vi "EditValue.vi"(8 "error in (no error)":errorcluster, 10 "Bounds":T1, 11 "Floating point base in":refnum<class "Floating point base.lvclass">) -> (0 "error out":errorcluster, 1 "Tabbed out?":bool, 2 "Value changed?":bool, 3 "Floating point base out":refnum<class "Floating point base.lvclass">)   [LabVIEW 2018, in "D Datagrid Library.lvlib" / "Floating point base.lvclass"]
uses:
  Floating point base.lvclass
  <vilib>/Utility/miscctls.llb/LVRectTypeDef.ctl
  DatagridElement/DatagridElement.lvclass
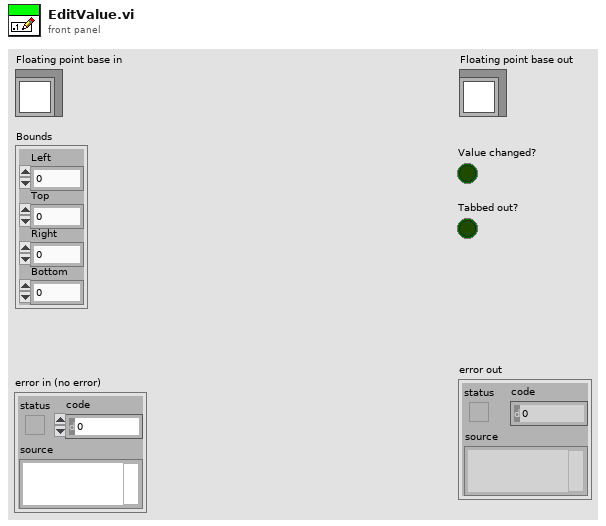
[diagram p1: front panel]
types:
  T1 = typedef "LVRectTypeDef.ctl" = cluster{"Left":i16, "Top":i16, "Right":i16, "Bottom":i16}
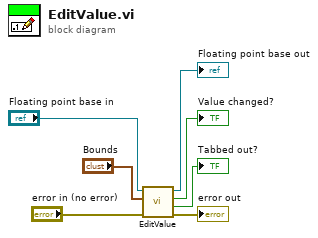
[diagram p0: block diagram]
diagram:
  n1 = call-parent "EditValue.vi"("error in (no error)"="error in (no error)", "Bounds"="Bounds", "DatagridElement in"="Floating point base in") -> ("error out"=→"error out":errorcluster, "Tabbed out?"=→"Tabbed out?":bool, "Value changed?"=→"Value changed?":bool, "DatagridElement out"=→"Floating point base out":refnum<class "Floating point base.lvclass">)  [unwired: 5 in]
